vi "Create.vi"(0 "Test Log Factory in":refnum<class "OperationsLogFactory.lvclass">, 5 "Test Log Types":T1, 7 "Test Name":string, 9 "Scan Name":string, 11 "error in (no error)":errorcluster) -> (4 "Test Log Factory out":refnum<class "OperationsLogFactory.lvclass">, 6 "Test Log":refnum<class "OperationsLog.lvclass">, 15 "error out":errorcluster)   [LabVIEW 2016, in "OperationsLogFactory.lvclass"]
uses:
  OperationsLogFactory.lvclass
  Test Log/OperationsLog.lvclass
  Typedefs/TestLogTypes.ctl
  common_configurationreader/ConfigurationReader.lvclass
  CSV Test Log/CSVOperationsLog.lvclass
  opt/CODE/ts_m1m3supporteui/Model/Test Log/Test Log/OperationsLog.lvclass
  Typedefs/LogPath.ctl
  Typedefs/M1M3SupportEUI_TypeDefs.lvlib
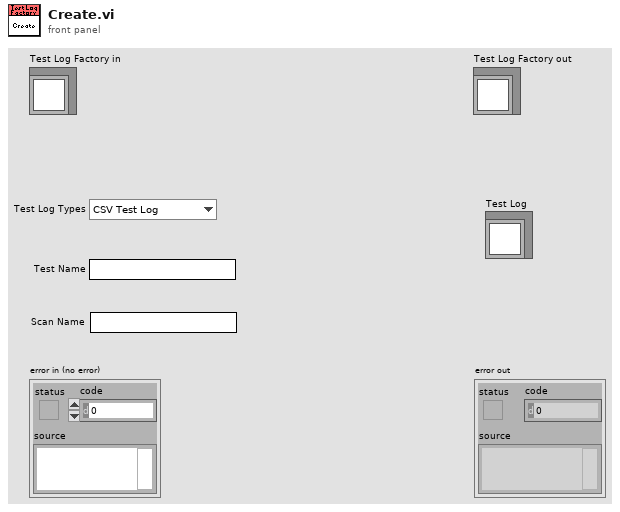
[diagram p1: front panel]
types:
  T1 = typedef "M1M3SupportEUI_TypeDefs.lvlib/TestLogTypes.ctl" = enum16{"CSV Test Log"}
  T2 = typedef "M1M3SupportEUI_TypeDefs.lvlib/LogPath.ctl" = path
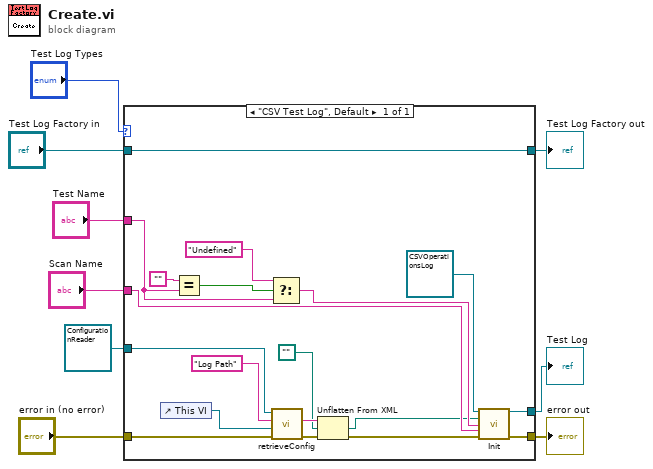
[diagram p0: block diagram]
diagram:
  n1 = case shown="\"CSV Test Log\", Default" "Test Log Types" {
    tunnel: "error in (no error)" -> [w23]
    tunnel: [w27] -> w3
    tunnel: [w18] -> w4
    tunnel: [w28] -> w2
    tunnel: "Test Log Factory in" -> [w28]
    tunnel: refnum<class "ConfigurationReader.lvclass"> refnum ("ConfigurationReader.lvclass") -> [w25]
    tunnel: "Test Name" -> [w15]
    tunnel: "Scan Name" -> [w12]
    frame "CSV Test Log", Default {
      n2 = control-ref of="This VI"() -> (w10:refnum<vi>)
      n3 = Equal?(x="", y=w15) -> (x = y?=w16:bool)
      n4 = Select(t="Undefined", s=w16, f=w15) -> (s? t:f=w14:string)
      n5 = call "retrieveConfig.vi"("error in (no error)"=w23, "callingVIRef"=w10, "configName"="Log Path", "ConfigurationReader in"=w25) -> ("error out"=w21:errorcluster, "xmlData"=w22:string)  [unwired: 5 in, 1 out]
      n6 = Unflatten From XML(xml string=w22, type=T2 path "" ("Log Path"), error in (no error)=w21) -> (value=w11:T2, error out=w19:errorcluster)
      n7 = call "Init.vi"("CSV Test Log in"=refnum<class "CSVOperationsLog.lvclass"> refnum ("CSVTestLog.lvclass"), "Log Path"=w11, "Test Name"=w14, "Scan Name"=w12, "error in (no error)"=w19) -> ("CSV Test Log out"=w27:refnum<class "CSVOperationsLog.lvclass">, "error out"=w18:errorcluster)  [unwired: 9 in]
    }
  }
  "error out" <- w4
  "Test Log Factory out" <- w2
  "Test Log" <- w3
